vi "SDR Fine Phase.vi"(0 "IVI Refnum in":refnum<k15>, 1 "Rm (ohm)":dbl, 2 "Step Size":cluster{"WLV":dbl, "BLV":dbl, "SLV":dbl}, 3 "MLC WLV (V)":dbl, 4 "MLC BLV (V)":dbl, 5 "error in (no error)":errorcluster, 6 "RM (ohm)":dbl, 7 "Initial resistance (ohm)":dbl, 8 "Max fine attempts":i32, 9 "MLC SLV (V)":dbl) -> (12 "target hit?":bool=TRUE, 13 "attempt number":i32=1, 14 "IVI Refnum out":refnum<k15>, 15 "Final resistance (ohm)":dbl, 16 "SL voltage (V)":dbl, 17 "BL voltage (V)":dbl, 18 "WL voltage (V)":dbl, 19 "error out":errorcluster)   [LabVIEW 2018]
uses:
  Globals.vi
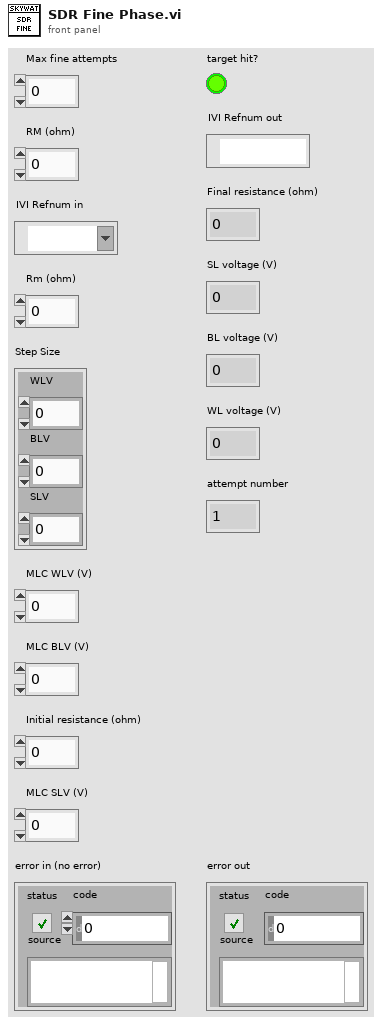
[diagram p1: front panel]
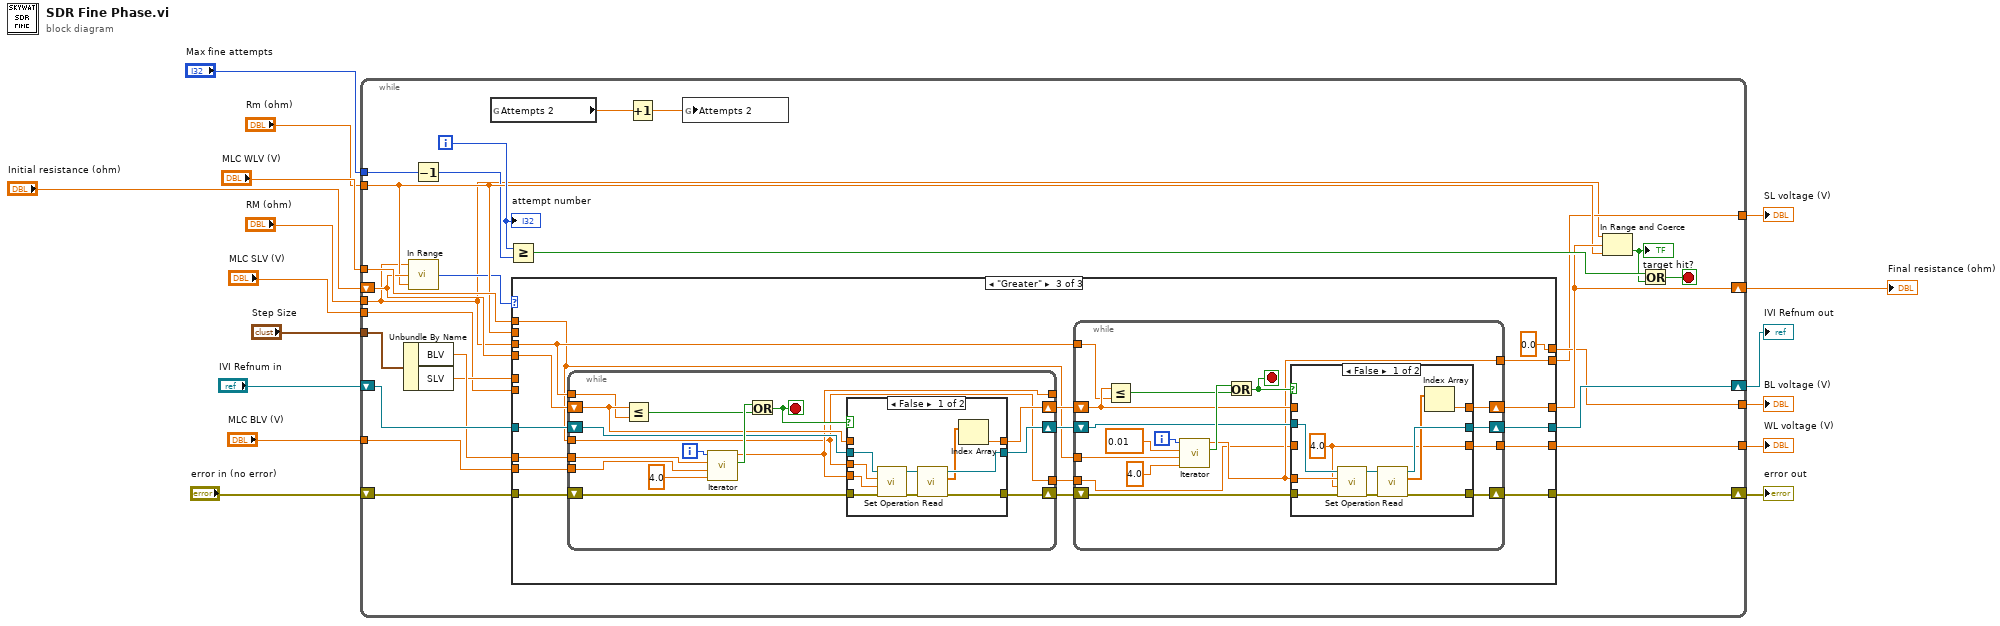
[diagram p0: block diagram]
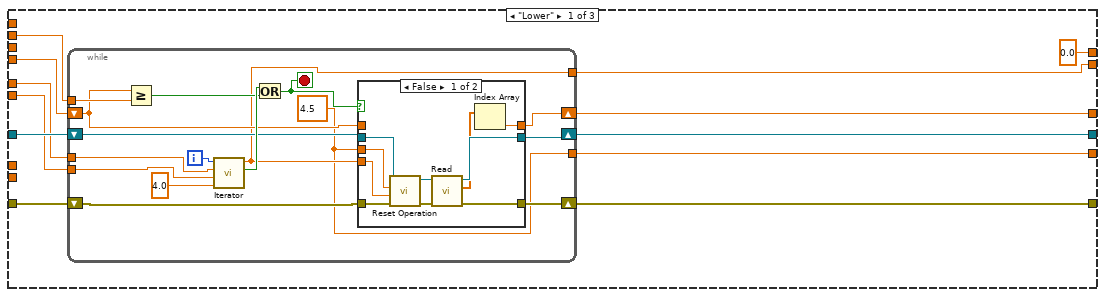
[diagram p2: hidden frame]
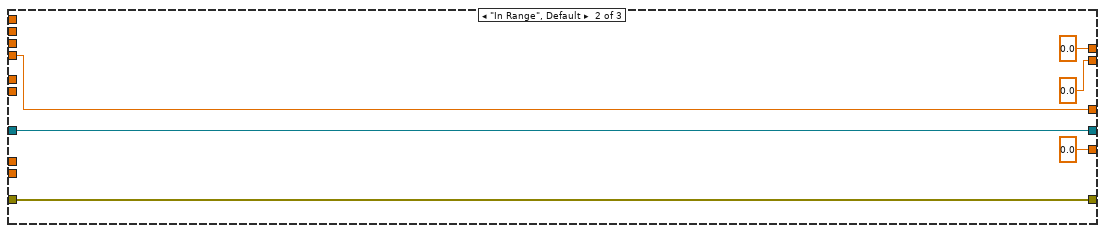
[diagram p4: hidden frame]
diagram:
  n1 = while {
    shift-right: [w37] -> w4
    shift-left: "IVI Refnum in" -> [w32]
    shift-right: [w36] -> w1
    shift-left: "error in (no error)" -> [w31]
    tunnel: "Max fine attempts" -> [w23]
    tunnel: "RM (ohm)" -> [w17]
    tunnel: "MLC WLV (V)" -> [w35]
    tunnel: "MLC BLV (V)" -> [w34]
    tunnel: "Rm (ohm)" -> [w30]
    tunnel: "Step Size" -> [w26]
    shift-right: [w38] -> w2
    shift-left: "Initial resistance (ohm)" -> [w33]
    tunnel: [w21] -> w13
    tunnel: [w20] -> w14
    tunnel: [w19] -> w15
    tunnel: "MLC SLV (V)" -> [w18]
    i -> [w41]
    stop <- w42 stop-if-true
    n2 = Unbundle By Name(w26) -> ("BLV"=w28:dbl, "SLV"=w27:dbl)
    n3 = call "In Range.vi"("Lower resistance (ohm)"=w30, "Resistance (ohm)"=w33, "Upper resistance (ohm)"=w17) -> ("range"=w29:enum16{"Lower", "In Range", "Greater"})
    n4 = Decrement(x=w23) -> (x-1=w22:i32)
    n5 = global read "Globals.vi" "Attempts 2"() -> (w24:dbl)
    n6 = Greater Or Equal?(x=w41, y=w22) -> (x >= y?=w40:bool)
    n7 = case shown="\"Greater\"" w29 {
      tunnel: w28 -> [_ _ w106]
      tunnel: w31 -> [w48 w88 w105]
      tunnel: [w52 w88 w98] -> w36
      tunnel: [w53 w89 w97] -> w37
      tunnel: [w47 w87 w99] -> w38
      tunnel: w17 -> [_ _ w93]
      tunnel: w32 -> [w50 w89 w104]
      tunnel: w33 -> [w51 w87 w103]
      tunnel: w30 -> [w54 _ _]
      tunnel: w35 -> [_ _ w90]
      tunnel: w34 -> [_ _ w102]
      tunnel: w27 -> [w49 _ _]
      tunnel: [w45 0.0 ("WL voltage (V)") w92] -> w21
      tunnel: [0.0 ("Current Value") 0.0 ("Current Value") 0.0 ("Current Value")] -> w20
      tunnel: [w44 0.0 ("Current Value") w100] -> w19
      tunnel: w18 -> [w46 _ _]
      frame "Lower" {
        n8 = while {
          shift-right: [w65] -> w53
          shift-left: w50 -> [w63]
          shift-right: [w66] -> w52
          shift-left: w48 -> [w64]
          tunnel: w54 -> [w61]
          shift-right: [w59] -> w47
          shift-left: w51 -> [w60]
          tunnel: w49 -> [w58]
          tunnel: [w57] -> w44
          tunnel: w46 -> [w56]
          tunnel: [w55] -> w45
          i -> [w70]
          stop <- w62 stop-if-true
          w55 = 4.5 ("WLV")
          n9 = Greater Or Equal?(x=w60, y=w61) -> (x >= y?=w67:bool)
          n10 = call "Iterator.vi"("Final Value"=4.0 ("y"), "Initial Value"=w56, "Step"=w58, "i"=w70) -> ("End Loop"=w68:bool, "Current Value"=w57:dbl)  [unwired: 6 in]
          n11 = Or(x=w68, y=w67) -> (x .or. y?=w62:bool)
          n12 = case shown="False" w62 {
            tunnel: w57 -> [w71 _]
            tunnel: [w78 w83] -> w66
            tunnel: [w77 w81] -> w65
            tunnel: w64 -> [w76 w83]
            tunnel: w63 -> [w75 w81]
            tunnel: w60 -> [_ w82]
            tunnel: [w73 w82] -> w59
            tunnel: w55 -> [w72 _]
            frame False {
              n13 = call "Reset Operation.vi"("error in (no error)"=w76, "SLV"=w71, "WLV"=w72, "instrument handle"=w75) -> ("error out"=w79:errorcluster, "instrument handle out"=w80:refnum<k15>)  [unwired: 6 in]
              n14 = call "Read.vi"("error in (no error)"=w79, "instrument handle"=w80) -> ("error out"=w78:errorcluster, "resistances (ohm)"=w74:dbl[], "instrument handle out"=w77:refnum<k15>)  [unwired: 6 in, 1 out]
              n15 = Index Array(array=w74) -> (element=w73:dbl)  [unwired: 1 in]
            }
            frame True {
            }
          }
        }
      }
      frame "In Range", Default {
      }
      frame "Greater" {
        n16 = while {
          shift-right: [w149] -> w96
          shift-left: w104 -> [w147]
          shift-right: [w150] -> w94
          shift-left: w105 -> [w148]
          tunnel: w93 -> [w141]
          tunnel: w106 -> [w145]
          shift-right: [w146] -> w95
          shift-left: w103 -> [w142]
          tunnel: w102 -> [w139]
          tunnel: [w140] -> _
          tunnel: [w138] -> w91
          tunnel: w90 -> [w138]
          i -> [w153]
          stop <- w144 stop-if-true
          n17 = Less Or Equal?(x=w142, y=w141) -> (x <= y?=w143:bool)
          n18 = call "Iterator.vi"("Final Value"=4.0 ("y"), "Initial Value"=w139, "Step"=w145, "i"=w153) -> ("End Loop"=w151:bool, "Current Value"=w140:dbl)  [unwired: 6 in]
          n19 = Or(x=w151, y=w143) -> (x .or. y?=w144:bool)
          n20 = case shown="False" w144 {
            tunnel: [w161 w166] -> w150
            tunnel: [w160 w164] -> w149
            tunnel: w140 -> [w159 _]
            tunnel: w148 -> [w158 w166]
            tunnel: w147 -> [w157 w164]
            tunnel: w142 -> [_ w165]
            tunnel: [w155 w165] -> w146
            tunnel: w138 -> [w154 _]
            frame False {
              n21 = call "Set Operation.vi"("error in (no error)"=w158, "BLV"=w159, "WLV"=w154, "instrument handle"=w157) -> ("error out"=w162:errorcluster, "instrument handle out"=w163:refnum<k15>)  [unwired: 6 in]
              n22 = call "Read.vi"("error in (no error)"=w162, "instrument handle"=w163) -> ("error out"=w161:errorcluster, "resistances (ohm)"=w156:dbl[], "instrument handle out"=w160:refnum<k15>)  [unwired: 6 in, 1 out]
              n23 = Index Array(array=w156) -> (element=w155:dbl)  [unwired: 1 in]
            }
            frame True {
            }
          }
        }
        n24 = while {
          shift-right: [w119] -> w97
          shift-left: w96 -> [w117]
          shift-right: [w120] -> w98
          shift-left: w94 -> [w118]
          shift-right: [w116] -> w99
          shift-left: w95 -> [w113]
          tunnel: [w109] -> w100
          tunnel: w93 -> [w112]
          tunnel: w90 -> [w111]
          tunnel: [w108] -> w92
          tunnel: w91 -> [w107]
          i -> [w123]
          stop <- w115 stop-if-true
          n25 = Less Or Equal?(x=w113, y=w112) -> (x <= y?=w114:bool)
          n26 = call "Iterator.vi"("Final Value"=4.0 ("y"), "Initial Value"=w111, "Step"=0.01, "i"=w123) -> ("End Loop"=w121:bool, "Current Value"=w109:dbl)  [unwired: 6 in]
          n27 = Or(x=w121, y=w114) -> (x .or. y?=w115:bool)
          n28 = case shown="False" w115 {
            tunnel: [w131 w137] -> w120
            tunnel: [w130 w135] -> w119
            tunnel: w118 -> [w129 w137]
            tunnel: w117 -> [w128 w135]
            tunnel: w113 -> [_ w136]
            tunnel: [w126 w136] -> w116
            tunnel: w109 -> [w125 _]
            tunnel: [w124 w134] -> w108
            tunnel: w107 -> [_ w134]
            frame False {
              w124 = 4.0 ("BLV")
              n29 = call "Set Operation.vi"("error in (no error)"=w129, "BLV"=w124, "WLV"=w125, "instrument handle"=w128) -> ("error out"=w132:errorcluster, "instrument handle out"=w133:refnum<k15>)  [unwired: 6 in]
              n30 = call "Read.vi"("error in (no error)"=w132, "instrument handle"=w133) -> ("error out"=w131:errorcluster, "resistances (ohm)"=w127:dbl[], "instrument handle out"=w130:refnum<k15>)  [unwired: 6 in, 1 out]
              n31 = Index Array(array=w127) -> (element=w126:dbl)  [unwired: 1 in]
            }
            frame True {
            }
          }
        }
      }
    }
    n32 = Increment(x=w24) -> (x+1=w25:dbl)
    n33 = global write "Globals.vi" "Attempts 2"(w25) -> ()
    n34 = In Range and Coerce(upper limit=w17, x=w38, lower limit=w30) -> (In Range?=w39:bool)  [unwired: 1 out]
    "target hit?" <- w39
    n35 = Or(x=w40, y=w39) -> (x .or. y?=w42:bool)
    "attempt number" <- w41
  }
  "SL voltage (V)" <- w15
  "BL voltage (V)" <- w14
  "WL voltage (V)" <- w13
  "IVI Refnum out" <- w4
  "Final resistance (ohm)" <- w2
  "error out" <- w1
